vi "usbpt104+usbTC-arduino control PWM (concurrent4).vi"(6 "RTD 1 Temp Input":dbl, 9 "PID":T1={"proportional gain (Kc)"=5.0, "integral time (Ti, min)"=0.0, "derivative time (Td, min)"=0.0}, 10 "PID Temp Setpoint":u16=13, 11 "Duty Cycle Period (ms)":u32=1000) -> (0 "Low Pulse Duration (ms)":dbl, 1 "High Pulse Duration (ms)":dbl, 2 "Duty Cycle (%)":dbl format="%.2f", 3 "PWM":dynamicdata(graph) caption="Square", 4 "CH1 Value":dbl(slide) max=10000.0 scale=0.8..800.0)   [LabVIEW 2015]
uses:
  <vilib>/addons/control/pid/pid.llb/PID (DBL).vi
  <vilib>/addons/control/pid/NI_PID_pid.lvlib
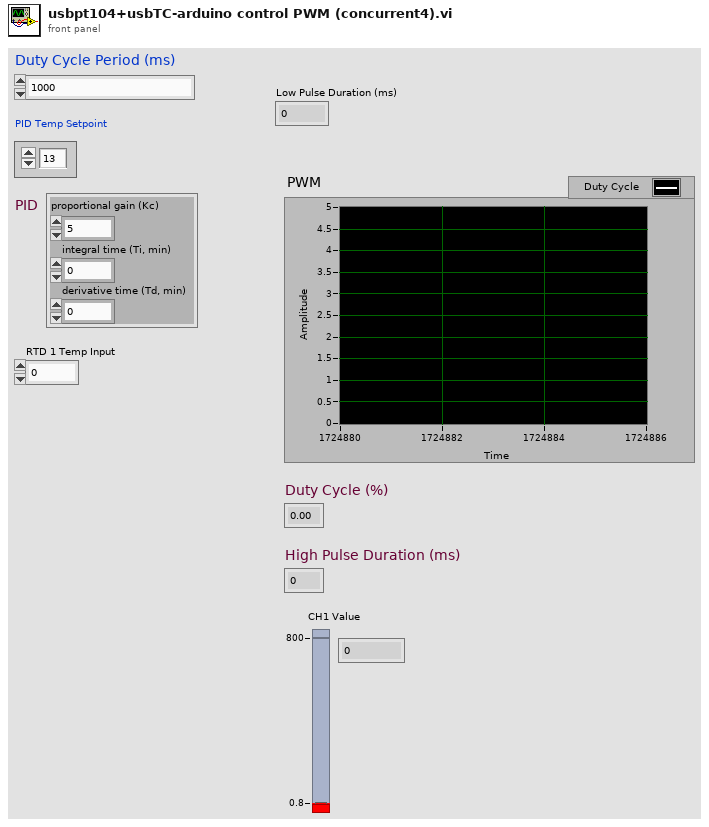
[diagram p1: front panel]
types:
  T1 = cluster{"proportional gain (Kc)":dbl, "integral time (Ti, min)":dbl, "derivative time (Td, min)":dbl}
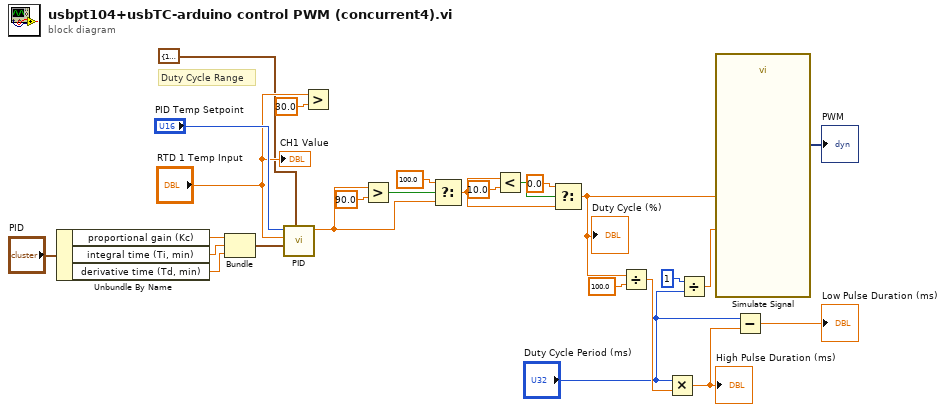
[diagram p0: block diagram]
diagram:
  # "Duty Cycle Range"
  n1 = Unbundle By Name("PID") -> ("proportional gain (Kc)"=w23:dbl, "integral time (Ti, min)"=w24:dbl, "derivative time (Td, min)"=w25:dbl)
  n2 = Bundle("proportional gain (Kc)"=w23, "integral time (Ti, min)"=w24, "derivative time (Td, min)"=w25) -> (w22:T1)  [unwired: 1 in]
  n3 = call-poly <vilib>:"PID.vi"("output range"=cluster{"output high":dbl, "output low":dbl} {"output high"=100.0, "output low"=0.0} ("Duty Cycle Range (%)"), "PID gains"=w22, "process variable"="RTD 1 Temp Input", "setpoint"="PID Temp Setpoint") -> ("output"=w20:dbl)  [unwired: 6 in, 1 out]
  n4 = Greater?(x="RTD 1 Temp Input", y=sgl 30.0) -> ()  [unwired: 1 out]
  n5 = Greater?(x=w20, y=90.0) -> (0:w8:bool)
  n6 = Select(t=100.0 ("f"), s=w8, f=w20) -> (s? t:f=w14:dbl)
  n7 = Less?(x=w14, y=10.0) -> (x < y?=w10:bool)
  n8 = Select(t=0.0 ("f"), s=w10, f=w14) -> (s? t:f=w19:dbl)
  "Duty Cycle (%)" <- w19
  n9 = Divide(x=w19, y=100.0) -> (x/y=w15:dbl)
  n10 = Multiply(x="Duty Cycle Period (ms)", y=w15) -> (x*y=w17:dbl)
  "High Pulse Duration (ms)" <- w17
  n11 = Divide(x=u32 1, y="Duty Cycle Period (ms)") -> (x/y=w6:dbl)
  n12 = call "Simulate Signal"("Duty Cycle (%)"=w19, "Frequency"=w6) -> ("Duty Cycle"=→"PWM":dynamicdata)  [unwired: 12 in, 1 out]
  n13 = Subtract(x="Duty Cycle Period (ms)", y=w17) -> (x-y=→"Low Pulse Duration (ms)":dbl)
  "CH1 Value" <- "RTD 1 Temp Input"
